vi "TeSAN.vi"() -> ()   [LabVIEW 2020]
uses:
  <vilib>/Instr/_visa.llb/VISA Configure Serial Port (Instr).vi
  <vilib>/Utility/file.llb/Write Delimited Spreadsheet (DBL).vi
panel:
  out "Piezo data":waveform(dbl)[](array[waveform])
  in  "Tab Control":enum32{"Piezo Sensor", "Motor Control"}(tab)
  in  "Radio Buttons":enum32{"RESET", "100pF", "10nF"}(radio)
  in  "정지":bool
  out "Waveform Chart":dynamicdata(graph)
  in  "rate":dbl=1000.0
  in  "number of samples":i32=100
  in  "G2":bool
  in  "G1":bool
  in  "G0":bool
  in  "100M":bool
  out "GAIN":i32=100
  out "Digital Signal indicatior":bool[](array[boolean])
  in  "Save Button":bool
  in  "Clear Button":bool
  out "XY Graph":cluster{dbl[], dbl[]}(graph)
  in  "VISA resource name":refnum<visa-resource-name>
  in  "baud rate":u32=9600
  out "read buffer":string
  out "Position":dbl
  out "LoadCell":dbl
  in  "TEST SETTING\n원위치":bool
  in  "TEST SETTING\n1초동안 위로 이동":bool
  in  "TEST SETTING\n0.5초동안 위로 이동":bool
  in  "TEST SETTING\n0.5초동안 아래로 이동":bool
  in  "TEST SETTING\nSET":bool
  in  "TEST SETTING\nedit box":string
  in  "Arduino OFF":bool
  in  "INITIALIZIND\nPOSITION":bool
  in  "INITIALIZING\nLOADCELL":bool
  in  "INITIALIZING\n+10":bool
  in  "INITIALIZING\n+100":bool
  in  "INITIALIZING\n+1000":bool
  in  "INITIALIZING\n-10":bool
  in  "INITIALIZING\n-100":bool
  in  "INITIALIZING\n-1000":bool
  in  "TEST SETTING\nON":bool
  in  "TEST SETTING\nOFF":bool
  in  "EMERGENCY":bool
  in  "TEST SETTING\n정지":bool
  in  "TEST SETTING\n1초동안 아래로 이동":bool
  # "INITIALIZING"
  # "TEST SETTING"
  # "kg"
  # "SENSOR INFORMATION"
  # "mm"
  # "N"
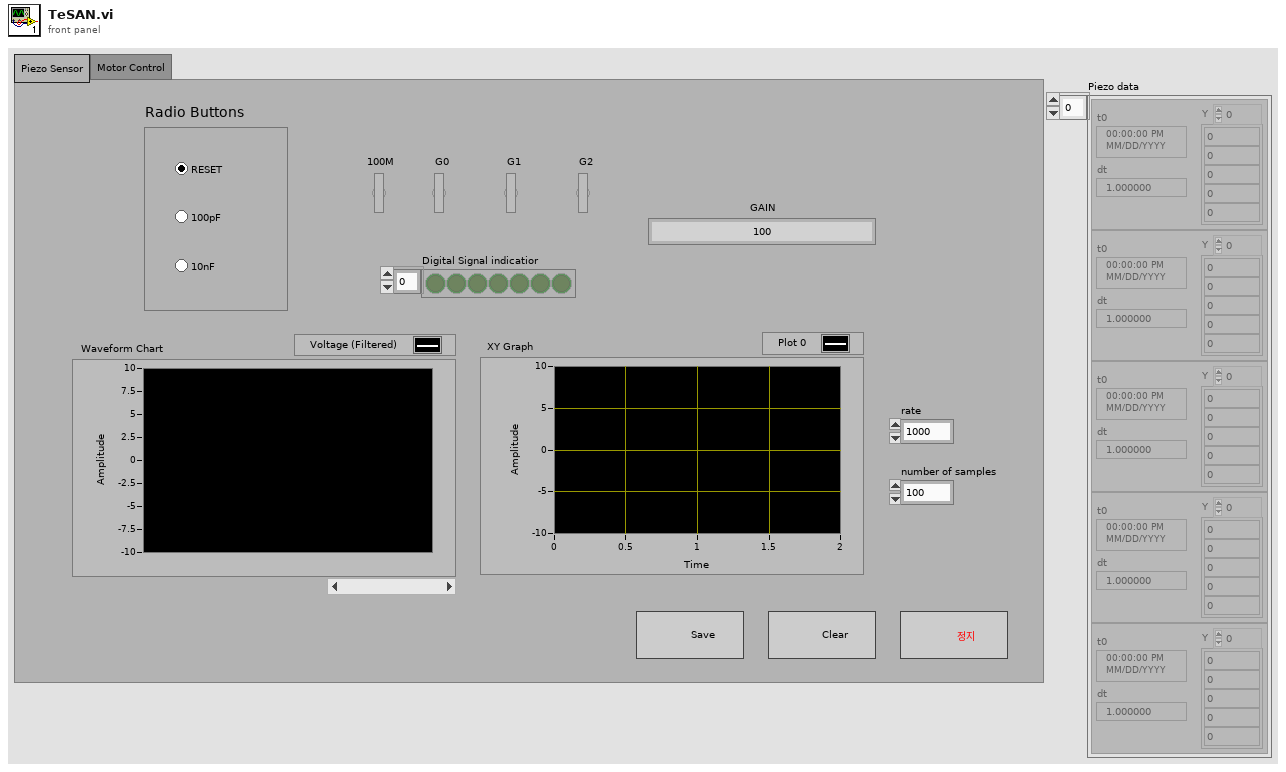
[diagram p1: front panel]
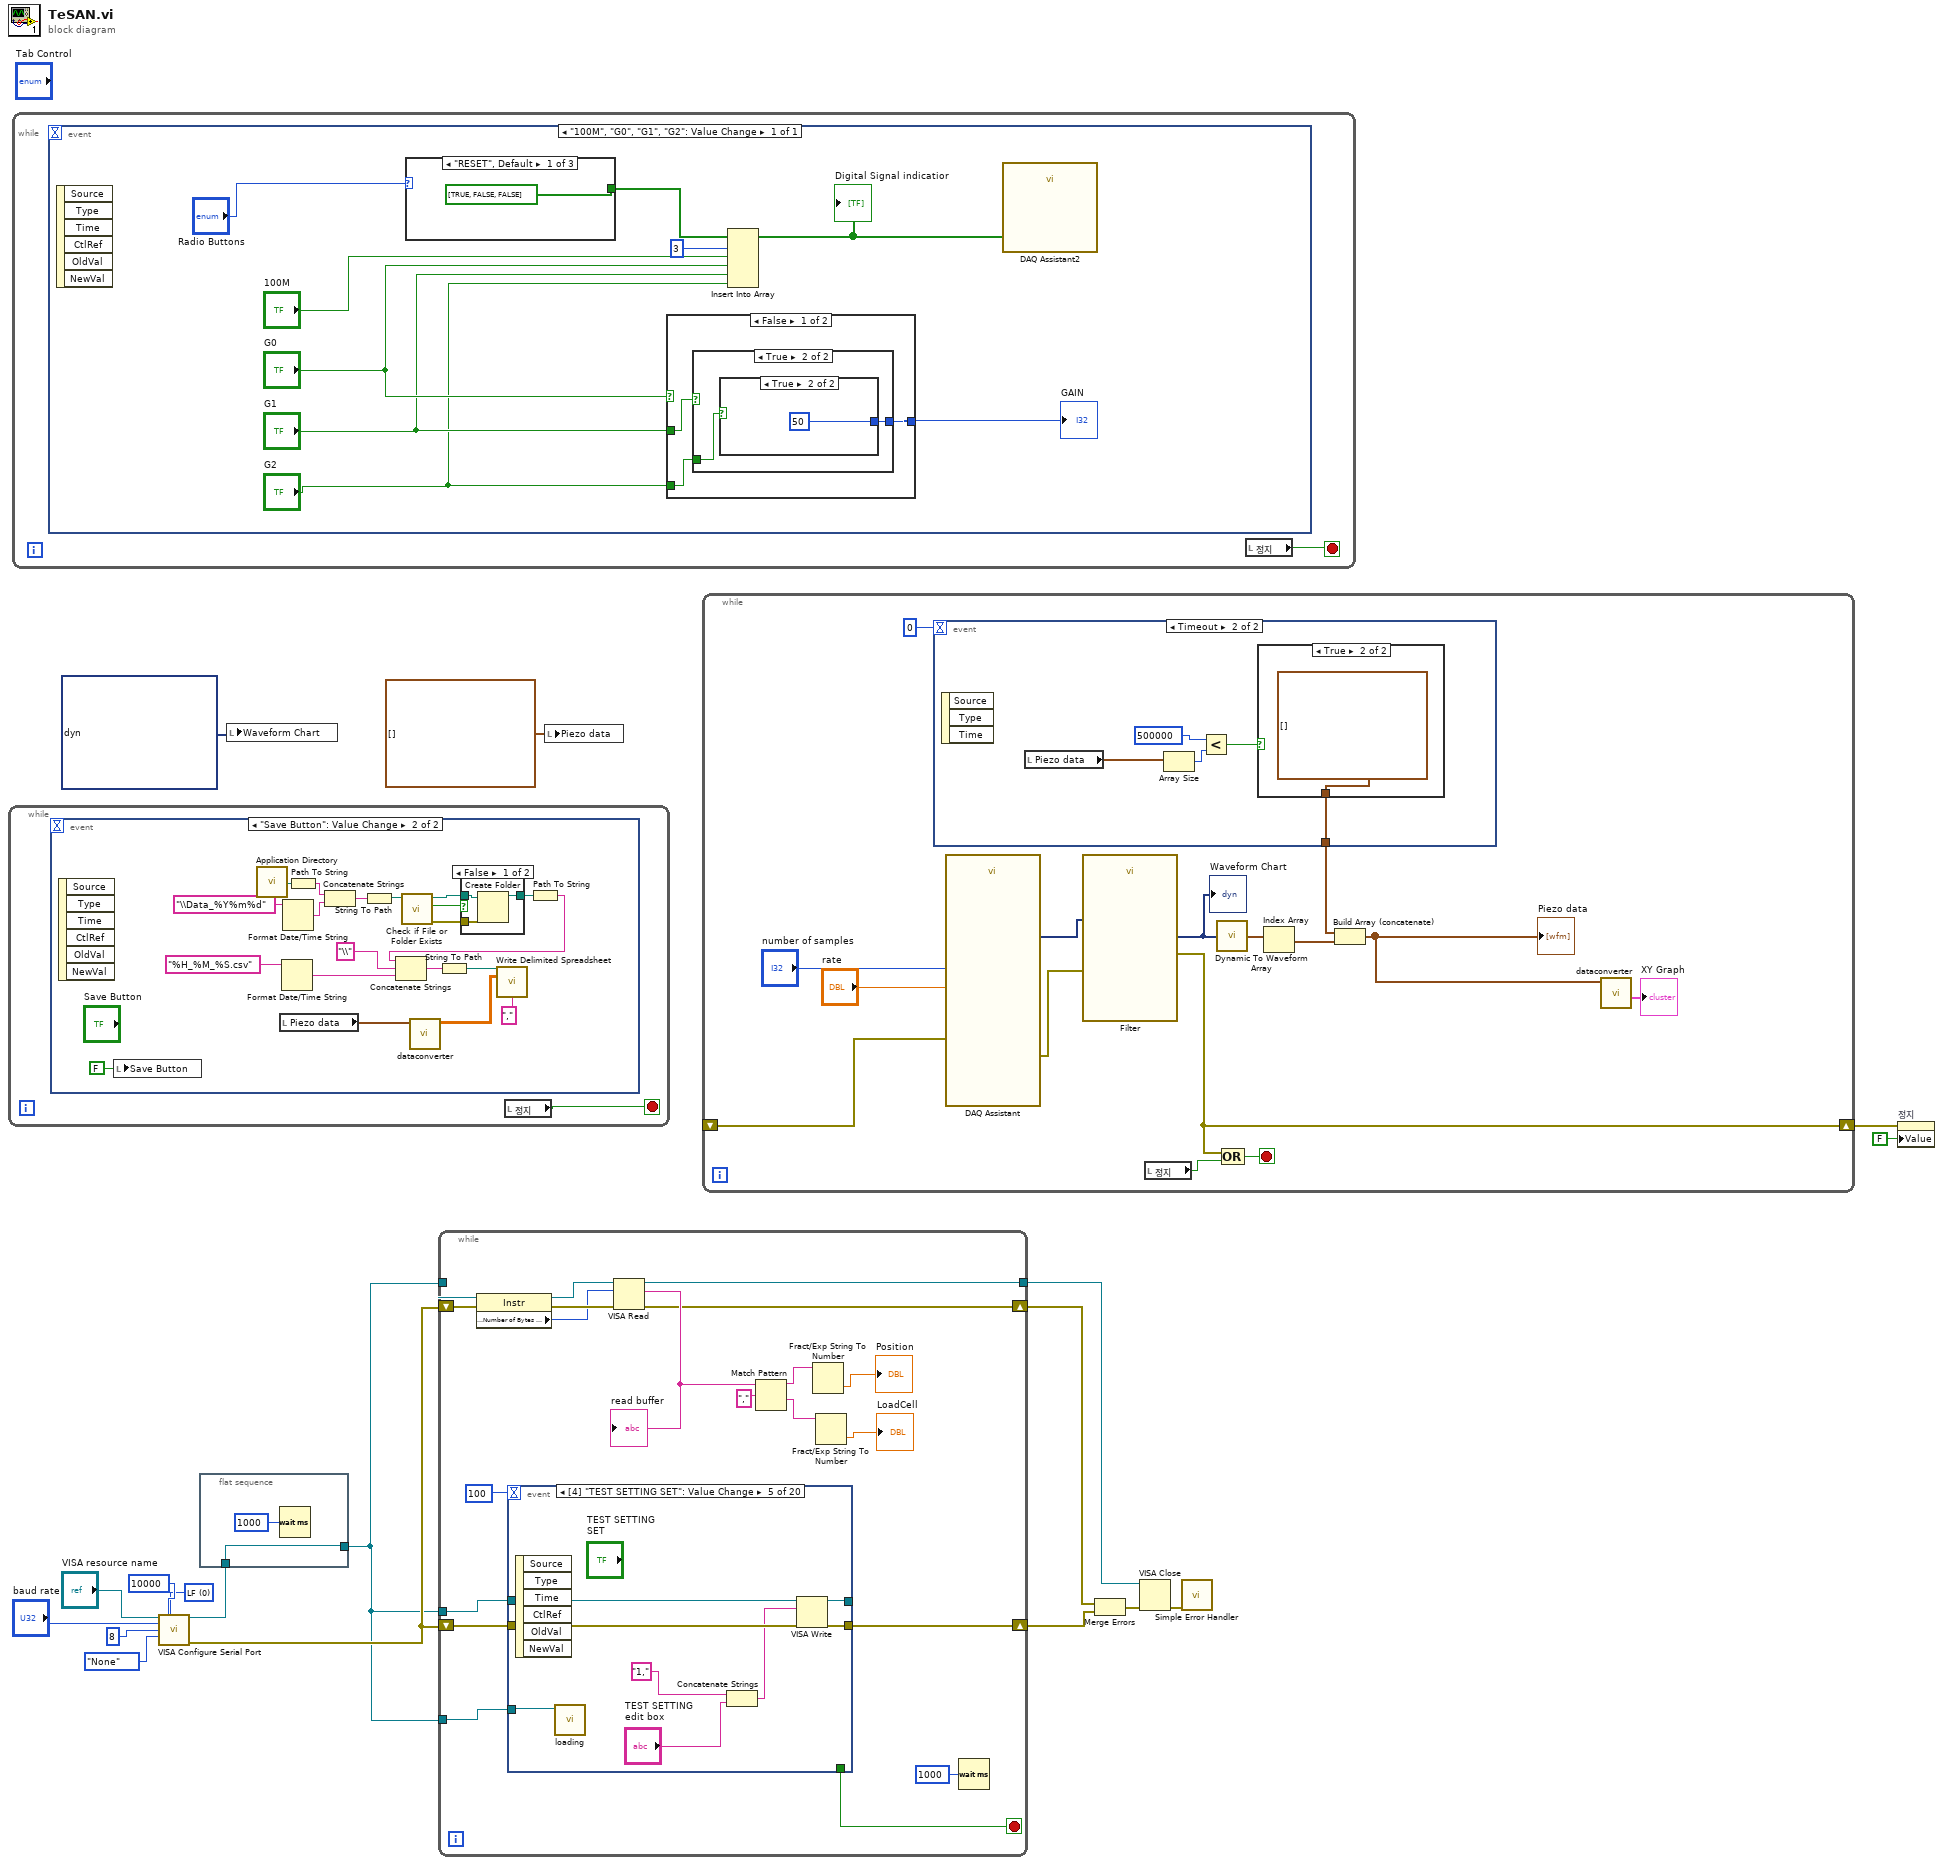
[diagram p0: block diagram]
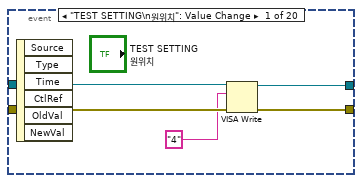
[diagram p2: hidden frame]
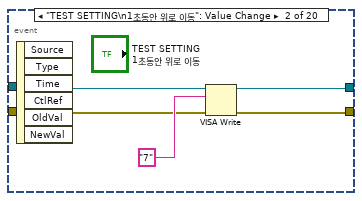
[diagram p3: hidden frame]
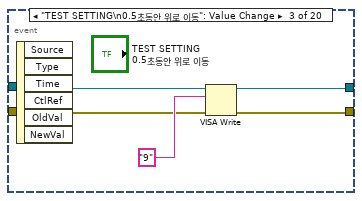
[diagram p4: hidden frame]
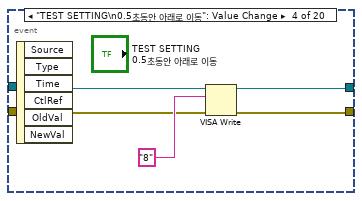
[diagram p5: hidden frame]
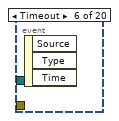
[diagram p6: hidden frame]
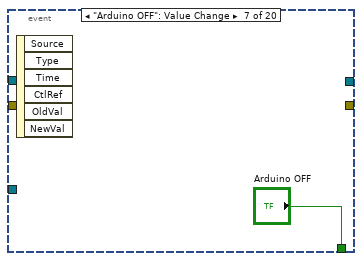
[diagram p7: hidden frame]
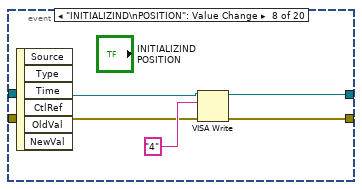
[diagram p8: hidden frame]
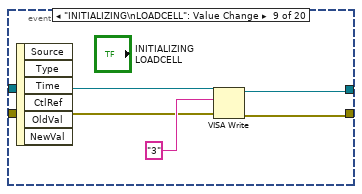
[diagram p9: hidden frame]
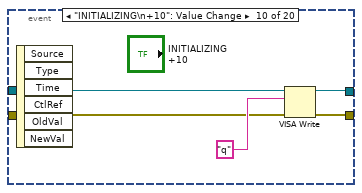
[diagram p10: hidden frame]
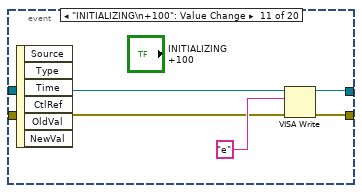
[diagram p11: hidden frame]
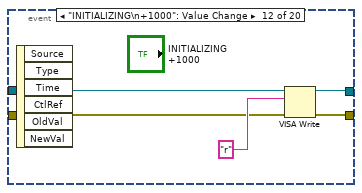
[diagram p12: hidden frame]
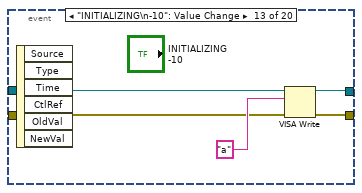
[diagram p13: hidden frame]
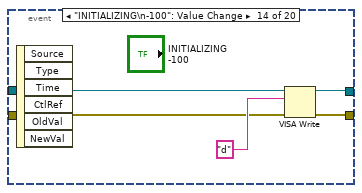
[diagram p14: hidden frame]
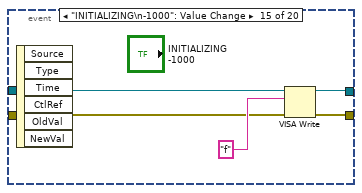
[diagram p15: hidden frame]
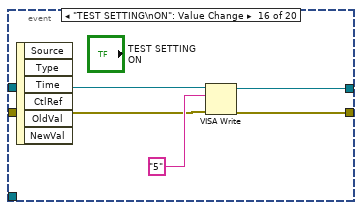
[diagram p16: hidden frame]
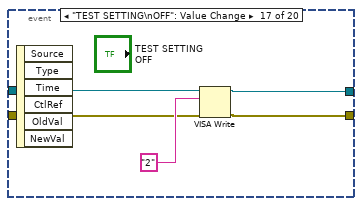
[diagram p17: hidden frame]
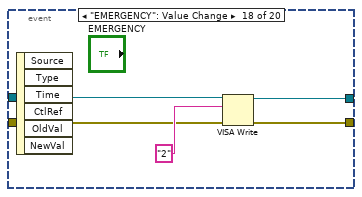
[diagram p18: hidden frame]
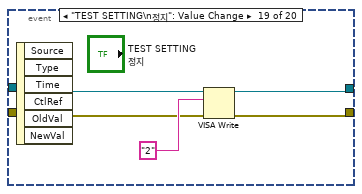
[diagram p19: hidden frame]
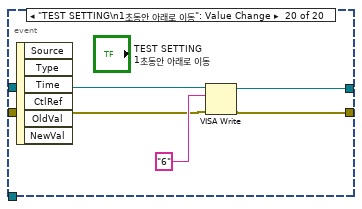
[diagram p20: hidden frame]
diagram:
  w3 = u16 0 items=["LF"]
  n1 = while {
    stop <- w19 stop-if-true
    n2 = event shown="[1] \"Save Button\": Value Change" {
      selector: _ -> [_ _]
      dyn-events: _ -> [_ _]
      timeout: _ -> [_ _]
      event "정지": Value Change {
        n3 = event-data() -> ()  [unwired: 1 in, 6 out]
      }
      event "Save Button": Value Change {
        n4 = event-data() -> ()  [unwired: 1 in, 6 out]
        n5 = local write "Save Button"(FALSE ("Save Button")) -> ()
        n6 = call <vilib>:"Application Directory.vi"() -> ("Application Directory"=w34:path)
        n7 = local read "Piezo data"() -> (w21:waveform(dbl)[])
        n8 = Format Date/Time String(time format string (%c)="%H_%M_%S.csv") -> (date/time string=w26:string)  [unwired: 2 in]
        n9 = Format Date/Time String(time format string (%c)="\\Data_%Y%m%d") -> (date/time string=w32:string)  [unwired: 2 in]
        n10 = Path To String(path=w34) -> (string=w33:string)
        n11 = Concatenate Strings(w33, w32) -> (w35:string)
        n12 = String To Path(string=w35) -> (path=w36:path)
        n13 = call <vilib>:"Check if File or Folder Exists.vi"("path"=w36) -> ("error out"=w37:errorcluster, "file or folder exists?"=w39:bool, "dup path"=w38:path)  [unwired: 8 in]
        n14 = call "dataconverter.vi"("appended array"=w21) -> ("transposed array"=w22:dbl[][])  [unwired: 9 in, 1 out]
        n15 = case shown="False" w39 {
          tunnel: w38 -> [w42 w43]
          tunnel: w37 -> [w41 _]
          tunnel: [w40 w43] -> w30
          frame False {
            n16 = Create Folder(path (use dialog)=w42, error in=w41) -> (created path=w40:path)  [unwired: 1 in, 2 out]
          }
          frame True {
          }
        }
        n17 = Path To String(path=w30) -> (string=w28:string)
        n18 = Concatenate Strings(w28, "\\" ("string"), w26) -> (w25:string)
        n19 = String To Path(string=w25) -> (path=w24:path)
        n20 = call-poly <vilib>:"Write Delimited Spreadsheet.vi"("file path (dialog if empty)"=w24, "2D data"=w22, "delimiter (\\t)"="," ("delimiter (\\t)")) -> ()  [unwired: 11 in, 2 out]
      }
    }
    n21 = local read "정지"() -> (w19:bool)
  }
  n22 = while {
    stop <- w44 stop-if-true
    n23 = event shown="[0] \"100M\", \"G0\", \"G1\", \"G2\": Value Change" {
      selector: _ -> [_]
      dyn-events: _ -> [_]
      timeout: _ -> [_]
      event "100M", "G0", "G1", "G2": Value Change {
        n24 = event-data() -> ()  [unwired: 1 in, 6 out]
        n25 = case shown="\"RESET\", Default" "Radio Buttons" {
          tunnel: [bool[] [TRUE, FALSE, FALSE] bool[] [FALSE, TRUE, FALSE] bool[] [FALSE, FALSE, TRUE]] -> w53
          frame "RESET", Default {
          }
          frame "100pF" {
          }
          frame "10nF" {
          }
        }
        n26 = case shown="False" "G0" {
          tunnel: [w56 w67] -> w50
          tunnel: "G1" -> [w55 w66]
          tunnel: "G2" -> [w54 w65]
          frame False {
            n27 = case shown="True" w55 {
              tunnel: [w58 w62] -> w56
              tunnel: w54 -> [w57 w61]
              frame False {
                n28 = case shown="False" w57 {
                  tunnel: [0 10] -> w58
                  frame False {
                  }
                  frame True {
                  }
                }
              }
              frame True {
                n29 = case shown="True" w61 {
                  tunnel: [2 50] -> w62
                  frame False {
                  }
                  frame True {
                  }
                }
              }
            }
          }
          frame True {
            n30 = case shown="False" w66 {
              tunnel: [w69 w73] -> w67
              tunnel: w65 -> [w68 w72]
              frame False {
                n31 = case shown="False" w68 {
                  tunnel: [1 20] -> w69
                  frame False {
                  }
                  frame True {
                  }
                }
              }
              frame True {
                n32 = case shown="False" w72 {
                  tunnel: [5 100] -> w73
                  frame False {
                  }
                  frame True {
                  }
                }
              }
            }
          }
        }
        "GAIN" <- w50
        n33 = Insert Into Array(array=w53, index=3, new element #1="100M", new element #2="G0", new element #3="G1", new element #4="G2") -> (w46:bool[])
        "Digital Signal indicatior" <- w46
        n34 = call "DAQ Assistant2"("data"=w46) -> ()  [unwired: 17 in, 2 out]
      }
    }
    n35 = local read "정지"() -> (w44:bool)
  }
  n36 = call-poly "VISA Configure Serial Port"("VISA resource name"="VISA resource name", "timeout (10sec)"=u32 10000, "termination char\n(0xA = '\\n' = LF)"=w3, "baud rate (9600)"="baud rate", "data bits (8)"=u16 8, "parity (0:none)"=enum16{"None", "Odd", "Even", "Mark", "Space"}."None") -> ("VISA resource name out"=w7:refnum<visa-resource-name>, "error out"=w14:errorcluster)  [unwired: 8 in]
  n37 = flat-sequence {
    tunnel: [w79] -> w13
    tunnel: w7 -> [w79]
    frame #0 {
      n38 = Wait (ms)(milliseconds to wait=u32 1000 ("대기 시간(ms)")) -> ()  [unwired: 1 out]
    }
  }
  n39 = local write "Waveform Chart"(dynamicdata [] ("Waveform Chart")) -> ()
  n40 = while {
    tunnel: w13 -> [w87]
    tunnel: w13 -> [w86]
    tunnel: [w83] -> w12
    tunnel: w13 -> [w81]
    shift-right: [w84] -> w11
    shift-left: w14 -> [w88]
    shift-right: [w85] -> w9
    shift-left: w14 -> [w89]
    stop <- w82 stop-if-true
    n41 = property class="Instr"(reference=w87, error in=w88) -> (reference out=w97:refnum<visa-resource-name>, error out=w98:errorcluster, "Serial Settings:Number of Bytes at Serial Port"=w96:u32)
    n42 = event shown="[4] \"TEST SETTING SET\": Value Change" {
      selector: _ -> [_ _ _ _ _ _ _ _ _ _ _ _ _ _ _ _ _ _ _ _]
      dyn-events: _ -> [_ _ _ _ _ _ _ _ _ _ _ _ _ _ _ _ _ _ _ _]
      timeout: 100 -> [_ _ _ _ _ _ _ _ _ _ _ _ _ _ _ _ _ _ _ _]
      tunnel: w89 -> [w105 w108 w113 w118 w127 _ _ w133 w137 w140 w145 w150 w155 w160 w165 w172 w177 w182 w187 w192]
      tunnel: w86 -> [w104 w109 w114 w119 w128 _ _ w132 w138 w141 w146 w151 w156 w161 w166 w173 w178 w183 w188 w193]
      tunnel: [w102 w106 w111 w116 w125 _ _ w130 w135 w142 w147 w152 w157 w162 w167 w170 w175 w180 w185 w190] -> w85
      tunnel: [w101 w107 w112 w117 w126 _ _ w131 w136 w143 w148 w153 w158 w163 w168 w171 w176 w181 w186 w191] -> _
      tunnel: w81 -> [_ _ _ _ w121 _ _ _ _ _ _ _ _ _ _ _ _ _ _ _]
      tunnel: [_ _ _ _ _ _ "Arduino OFF" _ _ _ _ _ _ _ _ _ _ _ _ _] -> w82
      event "TEST SETTING\n원위치": Value Change {
        n43 = event-data() -> ()  [unwired: 1 in, 6 out]
        n44 = VISA Write(VISA resource name=w104, write buffer="4", error in (no error)=w105) -> (VISA resource name out=w101:refnum<visa-resource-name>, error out=w102:errorcluster)  [unwired: 1 out]
      }
      event "TEST SETTING\n1초동안 위로 이동": Value Change {
        n45 = event-data() -> ()  [unwired: 1 in, 6 out]
        n46 = VISA Write(VISA resource name=w109, write buffer="7", error in (no error)=w108) -> (VISA resource name out=w107:refnum<visa-resource-name>, error out=w106:errorcluster)  [unwired: 1 out]
      }
      event "TEST SETTING\n0.5초동안 위로 이동": Value Change {
        n47 = event-data() -> ()  [unwired: 1 in, 6 out]
        n48 = VISA Write(VISA resource name=w114, write buffer="9", error in (no error)=w113) -> (VISA resource name out=w112:refnum<visa-resource-name>, error out=w111:errorcluster)  [unwired: 1 out]
      }
      event "TEST SETTING\n0.5초동안 아래로 이동": Value Change {
        n49 = event-data() -> ()  [unwired: 1 in, 6 out]
        n50 = VISA Write(VISA resource name=w119, write buffer="8", error in (no error)=w118) -> (VISA resource name out=w117:refnum<visa-resource-name>, error out=w116:errorcluster)  [unwired: 1 out]
      }
      event "TEST SETTING\nSET": Value Change {
        n51 = event-data() -> ()  [unwired: 1 in, 6 out]
        n52 = call "loading.vi"("VISA resource name"=w121) -> ()  [unwired: 11 in]
        n53 = Concatenate Strings("1," ("write buffer"), "TEST SETTING\nedit box") -> (w124:string)
        n54 = VISA Write(VISA resource name=w128, write buffer=w124, error in (no error)=w127) -> (VISA resource name out=w126:refnum<visa-resource-name>, error out=w125:errorcluster)  [unwired: 1 out]
      }
      event Timeout {
        n55 = event-data() -> ()  [unwired: 1 in, 3 out]
      }
      event "Arduino OFF": Value Change {
        n56 = event-data() -> ()  [unwired: 1 in, 6 out]
      }
      event "INITIALIZIND\nPOSITION": Value Change {
        n57 = event-data() -> ()  [unwired: 1 in, 6 out]
        n58 = VISA Write(VISA resource name=w132, write buffer="4", error in (no error)=w133) -> (VISA resource name out=w131:refnum<visa-resource-name>, error out=w130:errorcluster)  [unwired: 1 out]
      }
      event "INITIALIZING\nLOADCELL": Value Change {
        n59 = event-data() -> ()  [unwired: 1 in, 6 out]
        n60 = VISA Write(VISA resource name=w138, write buffer="3", error in (no error)=w137) -> (VISA resource name out=w136:refnum<visa-resource-name>, error out=w135:errorcluster)  [unwired: 1 out]
      }
      event "INITIALIZING\n+10": Value Change {
        n61 = event-data() -> ()  [unwired: 1 in, 6 out]
        n62 = VISA Write(VISA resource name=w141, write buffer="q", error in (no error)=w140) -> (VISA resource name out=w143:refnum<visa-resource-name>, error out=w142:errorcluster)  [unwired: 1 out]
      }
      event "INITIALIZING\n+100": Value Change {
        n63 = event-data() -> ()  [unwired: 1 in, 6 out]
        n64 = VISA Write(VISA resource name=w146, write buffer="e", error in (no error)=w145) -> (VISA resource name out=w148:refnum<visa-resource-name>, error out=w147:errorcluster)  [unwired: 1 out]
      }
      event "INITIALIZING\n+1000": Value Change {
        n65 = event-data() -> ()  [unwired: 1 in, 6 out]
        n66 = VISA Write(VISA resource name=w151, write buffer="r", error in (no error)=w150) -> (VISA resource name out=w153:refnum<visa-resource-name>, error out=w152:errorcluster)  [unwired: 1 out]
      }
      event "INITIALIZING\n-10": Value Change {
        n67 = event-data() -> ()  [unwired: 1 in, 6 out]
        n68 = VISA Write(VISA resource name=w156, write buffer="a", error in (no error)=w155) -> (VISA resource name out=w158:refnum<visa-resource-name>, error out=w157:errorcluster)  [unwired: 1 out]
      }
      event "INITIALIZING\n-100": Value Change {
        n69 = event-data() -> ()  [unwired: 1 in, 6 out]
        n70 = VISA Write(VISA resource name=w161, write buffer="d", error in (no error)=w160) -> (VISA resource name out=w163:refnum<visa-resource-name>, error out=w162:errorcluster)  [unwired: 1 out]
      }
      event "INITIALIZING\n-1000": Value Change {
        n71 = event-data() -> ()  [unwired: 1 in, 6 out]
        n72 = VISA Write(VISA resource name=w166, write buffer="f", error in (no error)=w165) -> (VISA resource name out=w168:refnum<visa-resource-name>, error out=w167:errorcluster)  [unwired: 1 out]
      }
      event "TEST SETTING\nON": Value Change {
        n73 = event-data() -> ()  [unwired: 1 in, 6 out]
        n74 = VISA Write(VISA resource name=w173, write buffer="5", error in (no error)=w172) -> (VISA resource name out=w171:refnum<visa-resource-name>, error out=w170:errorcluster)  [unwired: 1 out]
      }
      event "TEST SETTING\nOFF": Value Change {
        n75 = event-data() -> ()  [unwired: 1 in, 6 out]
        n76 = VISA Write(VISA resource name=w178, write buffer="2", error in (no error)=w177) -> (VISA resource name out=w176:refnum<visa-resource-name>, error out=w175:errorcluster)  [unwired: 1 out]
      }
      event "EMERGENCY": Value Change {
        n77 = event-data() -> ()  [unwired: 1 in, 6 out]
        n78 = VISA Write(VISA resource name=w183, write buffer="2", error in (no error)=w182) -> (VISA resource name out=w181:refnum<visa-resource-name>, error out=w180:errorcluster)  [unwired: 1 out]
      }
      event "TEST SETTING\n정지": Value Change {
        n79 = event-data() -> ()  [unwired: 1 in, 6 out]
        n80 = VISA Write(VISA resource name=w188, write buffer="2", error in (no error)=w187) -> (VISA resource name out=w186:refnum<visa-resource-name>, error out=w185:errorcluster)  [unwired: 1 out]
      }
      event "TEST SETTING\n1초동안 아래로 이동": Value Change {
        n81 = event-data() -> ()  [unwired: 1 in, 6 out]
        n82 = VISA Write(VISA resource name=w193, write buffer="6", error in (no error)=w192) -> (VISA resource name out=w191:refnum<visa-resource-name>, error out=w190:errorcluster)  [unwired: 1 out]
      }
    }
    n83 = VISA Read(VISA resource name=w97, byte count=w96, error in (no error)=w98) -> (VISA resource name out=w83:refnum<visa-resource-name>, read buffer=w99:string, error out=w84:errorcluster)  [unwired: 1 out]
    "read buffer" <- w99
    n84 = Match Pattern(string=w99, regular expression="," ("정규식")) -> (before substring=w94:string, after substring=w92:string)  [unwired: 1 in, 2 out]
    n85 = Fract/Exp String To Number(string=w94) -> (number=→"Position":dbl)  [unwired: 3 in, 1 out]
    n86 = Fract/Exp String To Number(string=w92) -> (number=→"LoadCell":dbl)  [unwired: 3 in, 1 out]
    n87 = Wait (ms)(milliseconds to wait=u32 1000 ("대기 시간(ms)")) -> ()  [unwired: 1 out]
  }
  n88 = local write "Piezo data"(waveform(dbl)[] [] ("Piezo data")) -> ()
  n89 = while {
    shift-right: [w203] -> w18
    shift-left: _ -> [w202]
    stop <- w204 stop-if-true
    n90 = event shown="[1] Timeout" {
      selector: _ -> [_ _]
      dyn-events: _ -> [_ _]
      timeout: 0 -> [_ _]
      tunnel: [waveform(dbl)[] [] ("Piezo data") w212] -> w198
      event "Clear Button": Value Change {
        n91 = event-data() -> ()  [unwired: 1 in, 6 out]
        n92 = local write "Clear Button"(FALSE ("Clear Button")) -> ()
      }
      event Timeout {
        n93 = event-data() -> ()  [unwired: 1 in, 3 out]
        n94 = local read "Piezo data"() -> (w213:waveform(dbl)[])
        n95 = Array Size(array=w213) -> (size(s)=w215:i32)
        n96 = Less?(x=500000, y=w215) -> (x < y?=w216:bool)
        n97 = case shown="True" w216 {
          tunnel: [w217 waveform(dbl)[] [] ("Piezo data")] -> w212
          frame False {
            n98 = local read "Piezo data"() -> (w217:waveform(dbl)[])
          }
          frame True {
          }
        }
      }
    }
    n99 = call "DAQ Assistant"("rate"="rate", "number of samples"="number of samples", "error in"=w202) -> ("data"=w207:dynamicdata, "error out"=w206:errorcluster)  [unwired: 13 in, 2 out]
    n100 = call "Filter"("error in (no error)"=w206, "Signal"=w207) -> ("error out"=w203:errorcluster, "Filtered Signal"=w197:dynamicdata)  [unwired: 8 in]
    "Waveform Chart" <- w197
    n101 = local read "정지"() -> (w205:bool)
    n102 = call <vilib>:"Dynamic To Waveform Array.vi"("Input"=w197) -> ("Output"=w201:waveform(dbl)[])  [unwired: 4 in]
    n103 = Compound Arithmetic op=OR(w203, w205) -> (w204:bool)
    n104 = Index Array(array=w201) -> (element=w200:waveform(dbl))  [unwired: 1 in]
    n105 = Build Array (concatenate)(w198, w200) -> (w195:waveform(dbl)[])
    "Piezo data" <- w195
    n106 = call "dataconverter.vi"("appended array"=w195) -> ("XY Graph"=→"XY Graph":cluster{dbl[], dbl[]})  [unwired: 9 in, 1 out]
  }
  n107 = Merge Errors(w11, w9) -> (w10:errorcluster)
  n108 = VISA Close(VISA resource name=w12, error in (no error)=w10) -> (error out=w8:errorcluster)
  n109 = call <vilib>:"Simple Error Handler.vi"("error in (no error)"=w8) -> ()  [unwired: 4 in, 5 out]
  n110 = property on="정지" class="Bool (strict)"(error in=w18, "Value"=FALSE ("stop")) -> ()  [unwired: 1 in, 2 out]
